vi "MultiScale SubVI.vi"(8 "error in (no error)":errorcluster, 10 "Image Dst":T1, 11 "Image Src":T1) -> (0 "error out":errorcluster, 2 "Pyr Levels":i32, 3 "Image Dst Out":T1)   [LabVIEW 2023]
uses:
  <vilib>/vision/Image Controls.llb/IMAQ Image.ctl
  <vilib>/vision/NI_Vision_Development_Module.lvlib
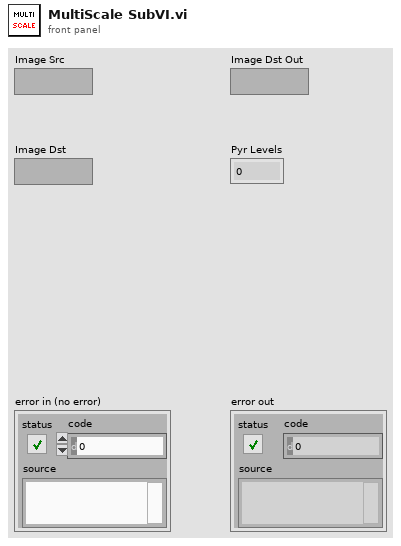
[diagram p1: front panel]
types:
  T1 = typedef "IMAQ Image.ctl" = refnum<image>
  T2 = typedef "Image Type" = u32
  T3 = typedef "Multiscale Parameters Typedef.ctl" = cluster{"Preprocessing":enum32{"Do Not Process", "Convolution", "Unsharp Mask"}, "Convolution":T4, "Unsharp Mask Params":T5, "LUT Power":sgl[], "LUT Multiplier":sgl[], "Filters":T4[], "X Value PostProc":sgl}
  T4 = typedef "Conv Flt Presets.ctl" = enum16{"None", "Seifert 5x5", "Seifert 7x7", "High Pass 5x5 ", "High Pass 7x7", "Highlight Details 3x3", "Highlight Details 5x5", "Highlight Detail 7x7"}
  T5 = typedef "Unsharp Mask Params TypeDef.ctl" = cluster{"Amount":sgl, "Radius":sgl, "Threshold":sgl}
  T6 = enum32{"Do Not Process", "Convolution", "Unsharp Mask"}
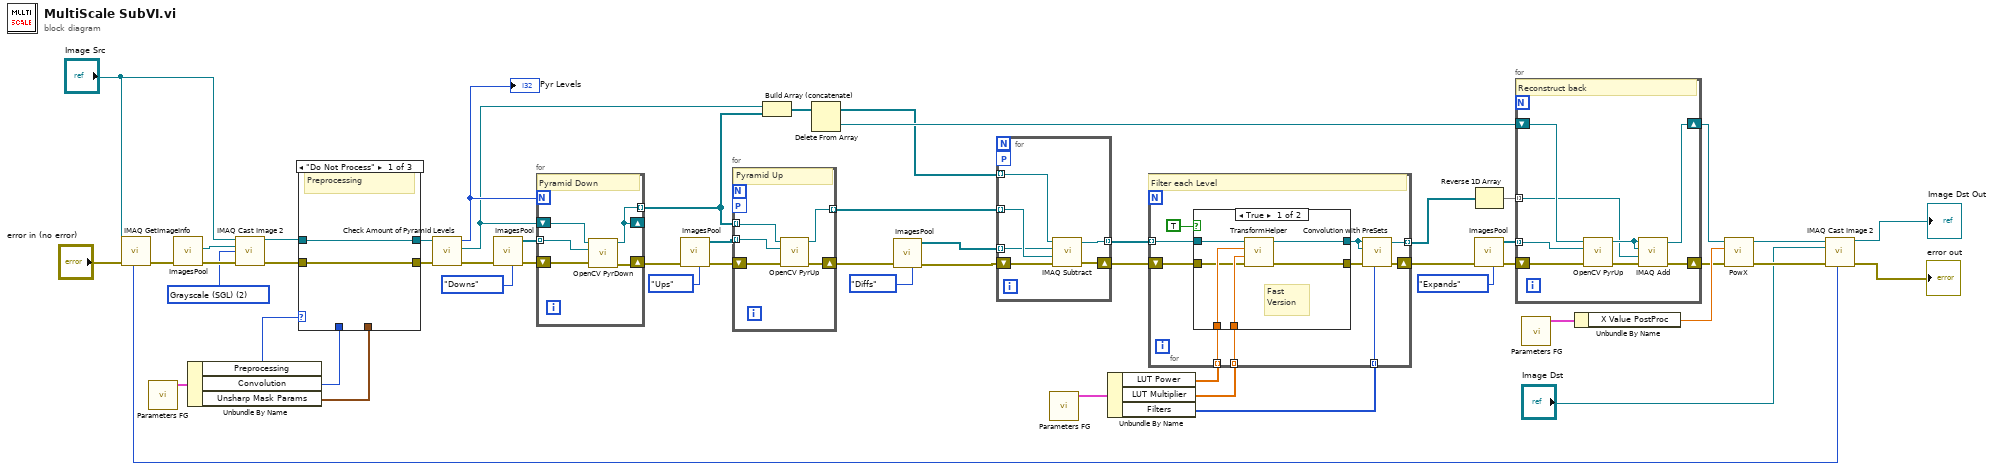
[diagram p0: block diagram]
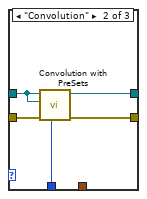
[diagram p2: hidden frame]
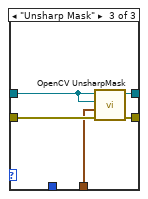
[diagram p3: hidden frame]
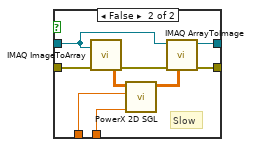
[diagram p4: hidden frame]
diagram:
  w37 = T2 2 items=["Grayscale (U8)", "Grayscale (I16)", "Grayscale (SGL)", "Complex (CSG)", "RGB (U32)", "HSL (U32)", "RGB (U64)", "Grayscale (U16)"] ("Image Type")
  n1 = call "IMAQ GetImageInfo"("error in (no error)"="error in (no error)", "Image"="Image Src") -> ("error out"=w3:errorcluster, "Image Type"=w5:T2)  [unwired: 2 in, 6 out]
  n2 = call "Parameters FG.vi"() -> ("MultiScale Parameters Out"=w27:T3)  [unwired: 10 in, 1 out]
  n3 = call "ImagesPool.vi"("error in (no error)"=w3) -> ("error out"=w50:errorcluster, "Filtered Copy"=w38:T1)  [unwired: 8 in, 1 out]
  n4 = Unbundle By Name(w27) -> ("Preprocessing"=w28:T6, "Convolution"=w29:T4, "Unsharp Mask Params"=w30:T5)
  n5 = call "IMAQ Cast Image 2"("Image Src"="Image Src", "Image Dst"=w38, "Image Type"=w37, "error in (no error)"=w50) -> ("Image Dst Out"=w40:T1, "error out"=w39:errorcluster)  [unwired: 10 in]
  n6 = case shown="\"Do Not Process\"" w28 {
    tunnel: w40 -> [w57 w59 w63]
    tunnel: [w56 w62 w67] -> w18
    tunnel: [w57 w61 w66] -> w19
    tunnel: w39 -> [w56 w58 w65]
    tunnel: w29 -> [_ w60 _]
    tunnel: w30 -> [_ _ w64]
    frame "Do Not Process" {
      # "Preprocessing"
    }
    frame "Convolution" {
      n7 = call "Convolution with PreSets.vi"("Filter"=w60, "error in (no error)"=w58, "Image Dst"=w59, "Image Src"=w59) -> ("error out"=w62:errorcluster, "Image Dst Out"=w61:T1)  [unwired: 5 in, 1 out]
    }
    frame "Unsharp Mask" {
      n8 = call "OpenCV UnsharpMask.vi"("error in (no error)"=w65, "Unsharp Mask Params"=w64, "Image Dst"=w63, "Image Src"=w63) -> ("error out"=w67:errorcluster, "Image Dst Out"=w66:T1)  [unwired: 5 in, 1 out]
    }
  }
  n9 = call "Check Amount of Pyramid Levels.vi"("error in (no error)"=w18, "Refnum in"=w19) -> ("error out"=w43:errorcluster, "Image Dup"=w20:T1, "Pyr Levels"=w55:i32)  [unwired: 7 in]
  "Pyr Levels" <- w55
  n10 = call "ImagesPool.vi"("Image"=enum16{"Ups", "Downs", "Diffs", "Expands"}."Downs", "error in (no error)"=w43) -> ("error out"=w44:errorcluster, "Array of Images"=w23:T1[])  [unwired: 7 in, 1 out]
  n11 = for {
    N: w55 -> [_]
    shift-right: [w71] -> _
    shift-left: w20 -> [w72]
    tunnel: [w71] -> w15 mode=indexing
    shift-right: [w70] -> w41
    shift-left: w44 -> [w68]
    tunnel: w23 -> [w69] mode=indexing
    # "Pyramid Down"
    n12 = call "OpenCV PyrDown.vi"("error in (no error)"=w68, "Image Dst"=w69, "Image Src"=w72) -> ("error out"=w70:errorcluster, "Image Dst Out"=w71:T1)  [unwired: 7 in]
  }
  n13 = call "ImagesPool.vi"("Image"=enum16{"Ups", "Downs", "Diffs", "Expands"}."Ups", "error in (no error)"=w41) -> ("error out"=w42:errorcluster, "Array of Images"=w24:T1[])  [unwired: 7 in, 1 out]
  n14 = for {
    tunnel: [w77] -> w9 mode=indexing
    tunnel: w15 -> [w76] mode=indexing
    shift-right: [w75] -> w45
    shift-left: w42 -> [w73]
    workers-P: _ -> [_]
    tunnel: w24 -> [w74] mode=indexing
    # "Pyramid Up"
    n15 = call "OpenCV PyrUp.vi"("error in (no error)"=w73, "Image Dst"=w74, "Image Src"=w76) -> ("error out"=w75:errorcluster, "Image Dst Out"=w77:T1)  [unwired: 7 in]
  }
  n16 = Build Array (concatenate)(w20, w15) -> (w7:T1[])
  n17 = Delete From Array(array=w7) -> (deleted portion=w10:T1, array with subset deleted=w8:T1[])  [unwired: 2 in]
  n18 = call "ImagesPool.vi"("Image"=enum16{"Ups", "Downs", "Diffs", "Expands"}."Diffs", "error in (no error)"=w45) -> ("error out"=w1:errorcluster, "Array of Images"=w25:T1[])  [unwired: 7 in, 1 out]
  n19 = for {
    tunnel: w8 -> [w83] mode=indexing
    tunnel: w9 -> [w82] mode=indexing
    tunnel: [w81] -> w13 mode=indexing
    shift-right: [w80] -> w16
    shift-left: w1 -> [w78]
    workers-P: _ -> [_]
    tunnel: w25 -> [w79] mode=indexing
    n20 = call "IMAQ Subtract"("Image Src A"=w83, "Image Dst"=w79, "Image Src B"=w82, "error in (no error)"=w78) -> ("Image Dst Out"=w81:T1, "error out"=w80:errorcluster)  [unwired: 3 in]
  }
  n21 = call "Parameters FG.vi"() -> ("MultiScale Parameters Out"=w31:T3)  [unwired: 10 in, 1 out]
  n22 = Unbundle By Name(w31) -> ("LUT Power"=w32:sgl[], "LUT Multiplier"=w33:sgl[], "Filters"=w34:T4[])
  n23 = for {
    tunnel: w13 -> [w93] mode=indexing
    tunnel: [w92] -> w12 mode=indexing
    tunnel: w32 -> [w90] mode=indexing
    tunnel: w33 -> [w89] mode=indexing
    shift-right: [w86] -> w46
    shift-left: w16 -> [w87]
    tunnel: w34 -> [w85] mode=indexing
    # "Filter each Level"
    n24 = case shown="True" TRUE {
      tunnel: w93 -> [w99 w108]
      tunnel: [w95 w107] -> w91
      tunnel: w90 -> [w98 w104]
      tunnel: w89 -> [w97 w103]
      tunnel: [w94 w101] -> w88
      tunnel: w87 -> [w96 w100]
      frame True {
        # "Fast\nVersion"
        n25 = call "TransformHelper.vi"("error in (no error)"=w96, "Multiplier"=w97, "Power"=w98, "Image  in"=w99) -> ("error out"=w94:errorcluster, "Image out"=w95:T1)  [unwired: 5 in, 1 out]
      }
      frame False {
        # "Slow"
        n26 = call "IMAQ ImageToArray"("error in (no error)"=w100, "Image"=w108) -> ("Image Pixels (Float)"=w106:sgl[][], "error out"=w102:errorcluster)  [unwired: 2 in, 3 out]
        n27 = call "PowerX 2D SGL.vi"("Multiplier"=w103, "Power"=w104, "Signal In"=w106) -> ("Signal Out"=w105:sgl[][])  [unwired: 8 in]
        n28 = call "IMAQ ArrayToImage"("Image Pixels (Float)"=w105, "error in (no error)"=w102, "Image"=w108) -> ("error out"=w101:errorcluster, "Image Out"=w107:T1)  [unwired: 7 in]
      }
    }
    n29 = call "Convolution with PreSets.vi"("Filter"=w85, "error in (no error)"=w88, "Image Dst"=w91, "Image Src"=w91) -> ("error out"=w86:errorcluster, "Image Dst Out"=w92:T1)  [unwired: 5 in, 1 out]
  }
  n30 = call "ImagesPool.vi"("Image"=enum16{"Ups", "Downs", "Diffs", "Expands"}."Expands", "error in (no error)"=w46) -> ("error out"=w47:errorcluster, "Array of Images"=w26:T1[])  [unwired: 7 in, 1 out]
  n31 = Reverse 1D Array(array=w12) -> (reversed array=w11:T1[])
  n32 = for {
    shift-right: [w113] -> w14
    shift-left: w10 -> [w116]
    tunnel: w11 -> [w114] mode=indexing
    shift-right: [w110] -> w17
    shift-left: w47 -> [w112]
    tunnel: w26 -> [w109] mode=indexing
    # "Reconstruct back"
    n33 = call "OpenCV PyrUp.vi"("error in (no error)"=w112, "Image Dst"=w109, "Image Src"=w116) -> ("error out"=w111:errorcluster, "Image Dst Out"=w115:T1)  [unwired: 7 in]
    n34 = call "IMAQ Add"("Image Src A"=w115, "Image Dst"=w115, "Image Src B"=w114, "error in (no error)"=w111) -> ("Image Dst Out"=w113:T1, "error out"=w110:errorcluster)  [unwired: 3 in]
  }
  n35 = call "Parameters FG.vi"() -> ("MultiScale Parameters Out"=w35:T3)  [unwired: 10 in, 1 out]
  n36 = Unbundle By Name(w35) -> ("X Value PostProc"=w36:sgl)
  n37 = call "PowX.vi"("error in (no error)"=w17, "X Value"=w36, "Refnum in"=w14) -> ("error out"=w48:errorcluster, "Refnum out"=w21:T1)  [unwired: 7 in]
  n38 = call "IMAQ Cast Image 2"("Image Src"=w21, "Image Dst"="Image Dst", "Image Type"=w5, "error in (no error)"=w48) -> ("Image Dst Out"=→"Image Dst Out":T1, "error out"=→"error out":errorcluster)  [unwired: 10 in]
